vi "setPhase.vi"(7 "Channel":string="0", 8 "error in (no error)":errorcluster, 10 "Phase [°]":dbl, 11 "FgenNiPxi in":refnum<class "ArbNi.lvclass">) -> (0 "error out":errorcluster, 3 "FgenNiPxi out":refnum<class "ArbNi.lvclass">)   [LabVIEW 2023, in "ArbNi.lvclass"]
doc: "<b>Author:</b> Wolfgang\n<b>Description:</b> Set Output Phase in degree"
uses:
  ArbNi.lvclass
  ArbNi.lvclass/ArbNi.ctl
  Arb.lvclass
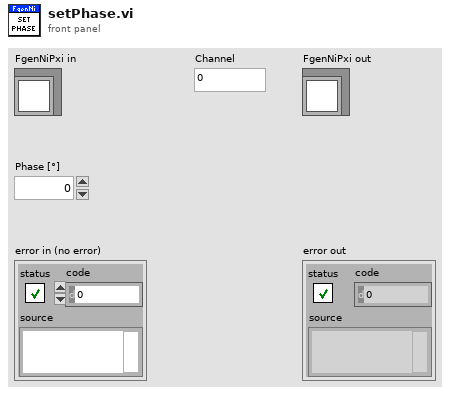
[diagram p1: front panel]
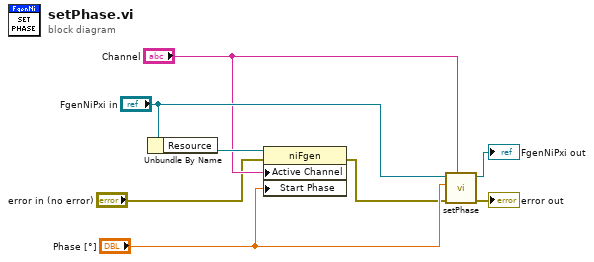
[diagram p0: block diagram]
diagram:
  n1 = Unbundle By Name("FgenNiPxi in") -> ("Resource"=w5:refnum<k15>)
  n2 = property class="niFgen"(reference=w5, error in="error in (no error)", "Active Channel"="Channel", "Start Phase"="Phase [°]") -> (error out=w1:errorcluster)  [unwired: 1 out]
  n3 = call-parent "setPhase.vi"("Channel"="Channel", "error in (no error)"=w1, "Phase [°]"="Phase [°]", "Fgen in"="FgenNiPxi in") -> ("error out"=→"error out":errorcluster, "Fgen out"=→"FgenNiPxi out":refnum<class "ArbNi.lvclass">)  [unwired: 6 in]
